vi "FieldDisp_Element_Rotate_Init.vi"(11 "Picture FIle Name":string) -> (0 "appended path":path, 1 "Height":i16, 2 "Width":i16, 3 "RotatedPictureInfo":T1)   [LabVIEW 2019, in "Trajectory_Library.lvlib"]
doc: "Internal function -- should not be called directly by users.\n\nComplete documentation TBD.\n\nInitialize a PNG image to be rotated."
uses:
  Trajectory_Library.lvlib
  TypeDef/FieldDisp_FieldElement.ctl
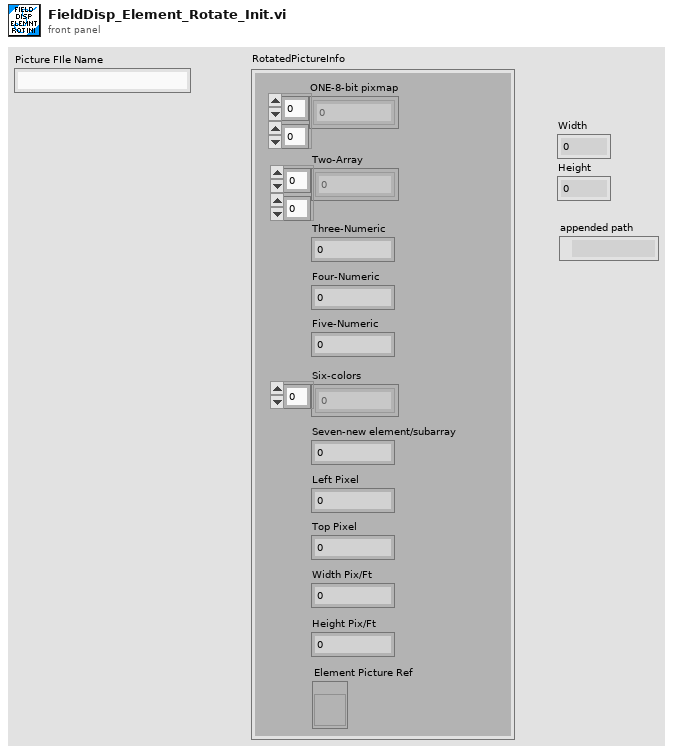
[diagram p1: front panel]
types:
  T1 = typedef "Trajectory_Library.lvlib/FieldDisp_FieldElement.ctl" = cluster{"ONE-8-bit pixmap":u8[][], "Two-Array":cdb[][], "Three-Numeric":i32, "Four-Numeric":i32, "Five-Numeric":cdb, "Six-colors":u32[], "Seven-new element/subarray":u32, "Left Pixel":dbl, "Top Pixel":dbl, "Width Pix/Ft":dbl, "Height Pix/Ft":dbl, "Element Picture Ref":refnum<vi>}
  T2 = typedef "imagedata.ctl" = cluster{"image type":i32, "image depth":i32, "image":u8[], "mask":u8[], "colors":u32[], "Rectangle":cluster{"left":i16, "top":i16, "right":i16, "bottom":i16}}
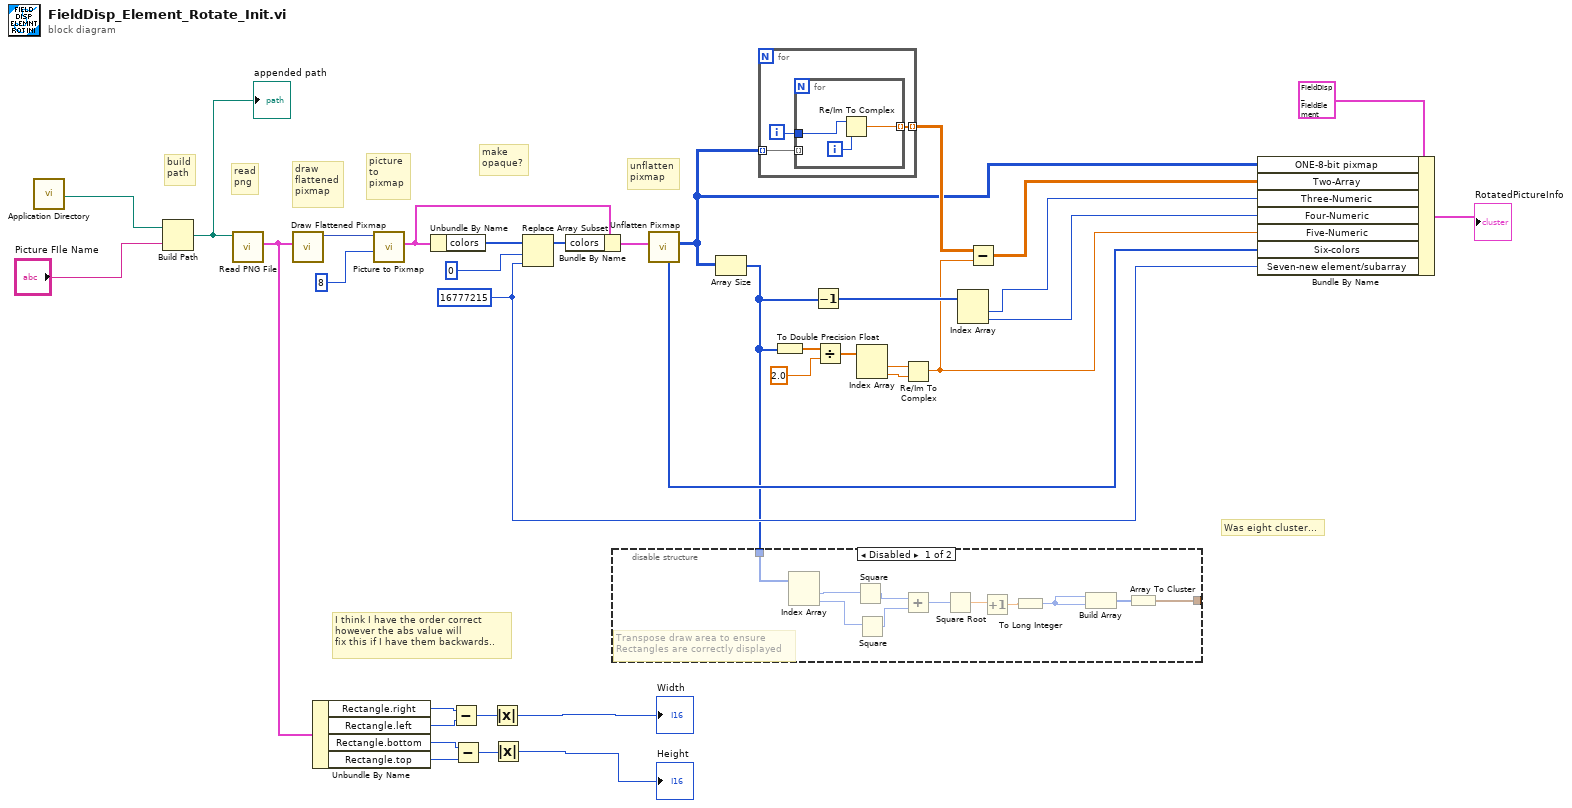
[diagram p0: block diagram]
diagram:
  w14 = u32 16777215 ("new element/subarray")
  # "Was eight cluster..."
  # "I think I have the order correct\nhowever the abs value will\nfix this if I have them backwards.."
  # "unflatten\npixmap"
  # "make\nopaque?"
  # "picture\nto\npixmap"
  # "draw\nflattened\npixmap"
  # "read\npng"
  # "build\npath"
  n1 = call <vilib>:"Application Directory.vi"() -> ("Application Directory"=w12:path)
  n2 = Build Path(base path=w12, name or relative path="Picture FIle Name") -> (appended path=w28:path)
  "appended path" <- w28
  n3 = call <vilib>:"Read PNG File.vi"("path to PNG file"=w28) -> ("image data"=w9:T2)  [unwired: 8 in, 2 out]
  n4 = call <vilib>:"Draw Flattened Pixmap.vi"("image data"=w9) -> ("new picture"=w33:picture)  [unwired: 8 in]
  n5 = Unbundle By Name(w9) -> ("Rectangle.right"=w8:i16, "Rectangle.left"=w7:i16, "Rectangle.bottom"=w6:i16, "Rectangle.top"=w5:i16)
  n6 = call <vilib>:"Picture to Pixmap.vi"("depth"=8, "picture"=w33) -> ("image data"=w35:T2)  [unwired: 8 in, 1 out]
  n7 = Unbundle By Name(w35) -> ("colors"=w30:u32[])
  n8 = Subtract(x=w8, y=w7) -> (x-y=w4:i16)
  n9 = Subtract(x=w6, y=w5) -> (x-y=w3:i16)
  n10 = Absolute Value(x=w4) -> (abs(x)=→"Width":i16)
  n11 = Absolute Value(x=w3) -> (abs(x)=→"Height":i16)
  n12 = Replace Array Subset(array=w30, new element=w14, index=0) -> (w32:u32[])
  n13 = Bundle By Name(cluster=w35, "colors"=w32) -> (w36:T2)
  n14 = call <vilib>:"Unflatten Pixmap.vi"("image data"=w36) -> ("8-bit pixmap"=w20:u8[][], "colors"=w15:u32[])  [unwired: 4 in, 5 out]
  n15 = Array Size(array=w20) -> (size(s)=w11:i32[])
  n16 = disable-structure shown="Disabled" {
    disable-tunnel: w11 -> [w47 _]
    disable-tunnel: [w37 _] -> _
    frame Disabled {
      # "Transpose draw area to ensure \nRectangles are correctly displayed"
      n17 = Index Array(array=w47) -> (element #1=w46:i32, element #2=w45:i32)  [unwired: 2 in]
      n18 = Square(x=w46) -> (x^2=w44:i32)
      n19 = Square(x=w45) -> (x^2=w43:i32)
      n20 = Add(x=w44, y=w43) -> (x+y=w42:i32)
      n21 = Square Root(x=w42) -> (sqrt(x)=w41:dbl)
      n22 = Increment(x=w41) -> (x+1=w40:dbl)
      n23 = To Long Integer(number=w40) -> (32bit integer=w39:i32)
      n24 = Build Array(w39, w39) -> (w38:i32[])
      n25 = Array To Cluster(array=w38) -> (cluster=w37:cluster{"[0]":i32, "[1]":i32})
    }
    frame Enabled {
    }
  }
  n26 = for {
    tunnel: [w49] -> w22 mode=indexing
    tunnel: w20 -> [w48] mode=indexing
    i -> [w50]
    n27 = for {
      tunnel: w50 -> [w53]
      tunnel: [w52] -> w49 mode=indexing
      tunnel: w48 -> [_] mode=indexing
      i -> [w51]
      n28 = Re/Im To Complex(1:w51, 2:w53) -> (0:w52:cdb)
    }
  }
  n29 = To Double Precision Float(number=w11) -> (double precision float=w10:dbl[])
  n30 = Decrement(x=w11) -> (x-1=w27:i32[])
  n31 = Divide(x=w10, y=2.0) -> (x/y=w24:dbl[])
  n32 = Index Array(array=w24) -> (element #1=w25:dbl, element #2=w26:dbl)  [unwired: 2 in]
  n33 = Re/Im To Complex(1:w26, 2:w25) -> (0:w16:cdb)
  n34 = Index Array(array=w27) -> (element #1=w18:i32, element #2=w17:i32)  [unwired: 2 in]
  n35 = Subtract(x=w22, y=w16) -> (x-y=w19:cdb[][])
  n36 = Bundle By Name(cluster=T1 {"ONE-8-bit pixmap"=[], "Two-Array"=[], "Three-Numeric"=0, "Four-Numeric"=0, "Five-Numeric"=0.0+0.0i, "Six-colors"=[], "Seven-new element/subarray"=0, "Left Pixel"=0.0, "Top Pixel"=0.0, "Width Pix/Ft"=0.0, "Height Pix/Ft"=0.0, "Element Picture Ref"=refnum} ("RotatedPictureInfo"), "ONE-8-bit pixmap"=w20, "Two-Array"=w19, "Three-Numeric"=w18, "Four-Numeric"=w17, "Five-Numeric"=w16, "Six-colors"=w15, "Seven-new element/subarray"=w14) -> (→"RotatedPictureInfo":T1)
